vi "VMI_set_date_path.vi"(0 "Value":path, 1 "Remote path 2":path, 2 "error in (no error)":errorcluster) -> (3 "appended path":path, 4 "New Date Name":string, 5 "appended path 2":path, 6 "error out":errorcluster)   [LabVIEW 2019]
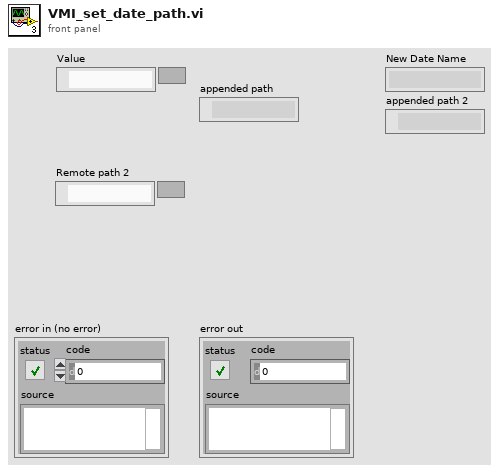
[diagram p1: front panel]
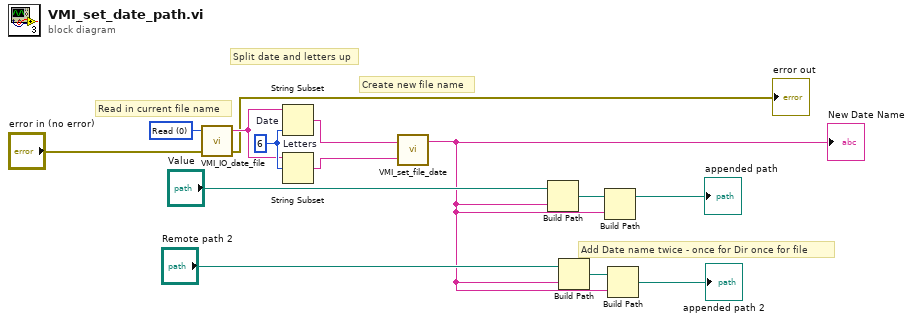
[diagram p0: block diagram]
diagram:
  w11 = 6 ("length (rest)")
  w9 = u16 0 items=["Read", "Write"] ("File Task")
  # "Add Date name twice - once for Dir once for file"
  # "Create new file name"
  # "Split date and letters up"
  # "Read in current file name"
  n1 = call "VMI_IO_date_file.vi"("Error In"="error in (no error)", "File Task"=w9) -> ("Error Out"=→"error out":errorcluster, "File date out"=w10:string)  [unwired: 2 in]
  n2 = String Subset "Date"(string=w10, length (rest)=w11) -> (substring=w12:string)  [unwired: 1 in]
  n3 = String Subset "Letters"(string=w10, offset (0)=w11) -> (substring=w13:string)  [unwired: 1 in]
  n4 = call "VMI_set_file_date.vi"("Saved date"=w12, "Ending"=w13) -> ("New Date Name"=w2:string)  [unwired: 2 out]
  "New Date Name" <- w2
  n5 = Build Path(base path="Value", name or relative path=w2) -> (appended path=w14:path)
  n6 = Build Path(base path="Remote path 2", name or relative path=w2) -> (appended path=w3:path)
  n7 = Build Path(base path=w14, name or relative path=w2) -> (appended path=→"appended path":path)
  n8 = Build Path(base path=w3, name or relative path=w2) -> (appended path=→"appended path 2":path)
